vi "Shooter PID.vi"(0 "Current RPM":dbl, 1 "Set RPM":dbl, 2 "Reinitialize?":bool) -> (7 "Motor":dbl format="%.2f")   [LabVIEW 2011]
uses:
  Team Code/Robot Global Data.vi
  <vilib>/addons/control/pid/pid.llb/PID (DBL).vi
  <vilib>/addons/control/pid/NI_PID_pid.lvlib
panel:
  in  "Allowable Error":dbl=15.0
  in  "1510 PID":T1={"proportional gain (Kc)"=1.0, "integral time (Ti, min)"=0.005, "derivative time (Td, min)"=0.0} {"derivative time (Td, min)" format="%.5f"; "integral time (Ti, min)" format="%.5f"; "proportional gain (Kc)" format="%.5f"}
  out "Error Graph":dbl(graph)
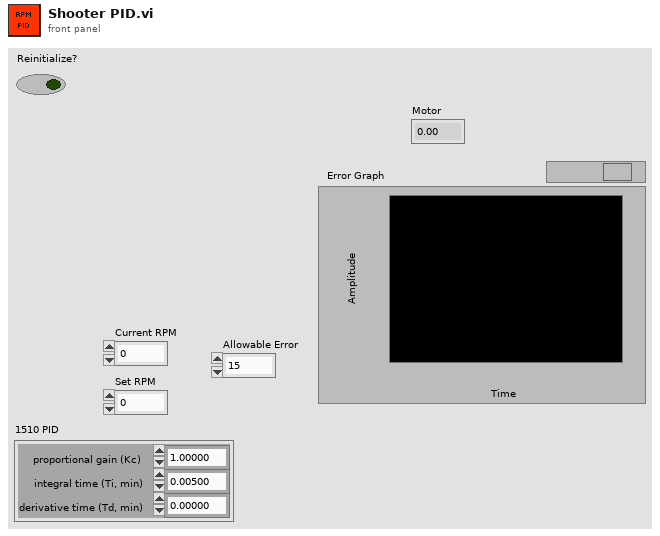
[diagram p1: front panel]
types:
  T1 = cluster{"proportional gain (Kc)":dbl, "integral time (Ti, min)":dbl, "derivative time (Td, min)":dbl}
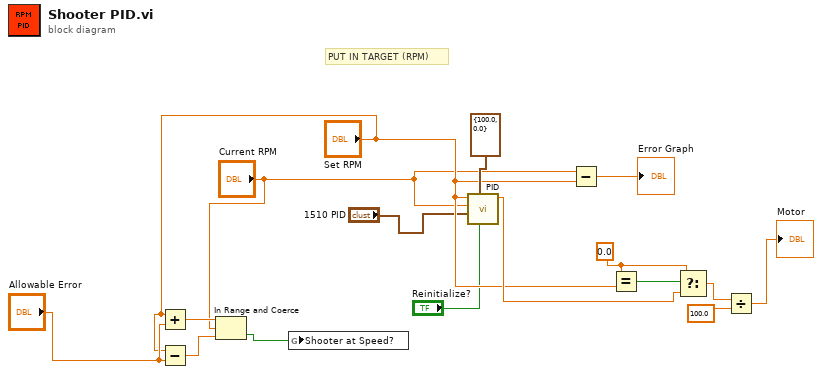
[diagram p0: block diagram]
diagram:
  w13 = 0.0 ("y")
  # "PUT IN TARGET (RPM)"
  n1 = Add(x="Set RPM", y="Allowable Error") -> (x+y=w7:dbl)
  n2 = Subtract(x="Set RPM", y="Allowable Error") -> (x-y=w8:dbl)
  n3 = In Range and Coerce(upper limit=w7, x="Current RPM", lower limit=w8) -> (In Range?=w3:bool)  [unwired: 1 out]
  n4 = global write "Robot Global Data.vi" "Shooter at Speed?"(w3) -> ()
  n5 = call-poly <vilib>:"PID.vi"("reinitialize? (F)"="Reinitialize?", "output range"=cluster{"output high":dbl, "output low":dbl} {"output high"=100.0, "output low"=0.0}, "PID gains"="1510 PID", "process variable"="Current RPM", "setpoint"="Set RPM") -> ("output"=w14:dbl)  [unwired: 5 in, 1 out]
  n6 = Subtract(x="Current RPM", y="Set RPM") -> (x-y=→"Error Graph":dbl)
  n7 = Equal?(x=w13, y="Set RPM") -> (x = y?=w15:bool)
  n8 = Select(t=w13, s=w15, f=w14) -> (s? t:f=w11:dbl)
  n9 = Divide(x=w11, y=100.0) -> (x/y=→"Motor":dbl)
